vi "실습 2-8 Home 찾기.vi"   [LabVIEW 2014]
uses:
  <vilib>/Motion/FlexMotion/CustomControls/CustomControls.llb/AxisOrVectorSpace To Control.flx
  <vilib>/Motion/FlexMotion/FunctionsVIs/Trajectory.llb/Check Move Complete Status (8 axes).flx
types:
  T1 = enum16{"Home", "Index", "Center", "Forward Limit", "Reverse Limit", "Run Sequence"}
  T2 = typedef "AxisOrVectorSpace To Control.flx" = u16
  T3 = typedef "Board Id" = u8
  T4 = typedef "Resource Out (Enum).flx" = u16
  T5 = typedef "Bd Id Out" = u8
  T6 = typedef "AxisOrVectorSpaceControl To Control.flx" = u16
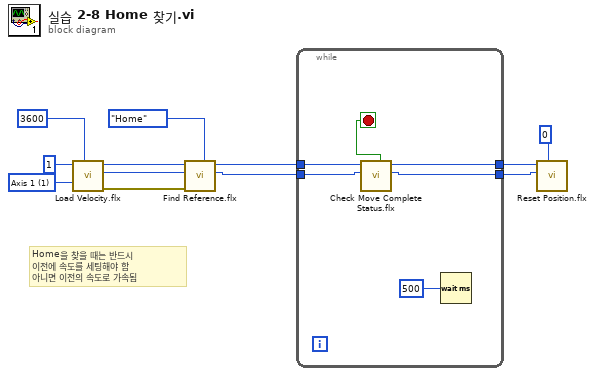
[diagram p0: block diagram]
diagram:
  w11 = T2 1 items=["Axis 1"=1, "Axis 2"=2, "Axis 3"=3, "Axis 4"=4, "Axis 5"=5, "Axis 6"=6, "Axis 7"=7, "Axis 8"=8, "Vector Space 1"=17, "Vector Space 2"=18, "Vector Space 3"=19, "Vector Space 4"=20] ("Axis or Vector Space")
  # "Home을 찾을 때는 반드시\n이전에 속도를 세팅해야 함\n아니면 이전의 속도로 가속됨"
  n1 = call <vilib>:"Load Velocity.flx"("Velocity (10000)"=3600, "Axis or Vector Space"=w11, "Board ID"=T3 1) -> ("error out"=w7:errorcluster, "Resource Output"=w8:T4, "Bd ID Out"=w9:T5)  [unwired: 4 in]
  n2 = call <vilib>:"Find Reference.flx"("Search Type"=T1."Home", "error in (no error)"=w7, "Axis or Vector Space"=w8, "Board ID"=w9) -> ("Axis or Vector Space Output"=w4:T6, "Bd ID Out"=w5:T5)  [unwired: 5 in, 1 out]
  n3 = while {
    tunnel: w5 -> [w18]
    tunnel: w4 -> [w17]
    tunnel: [w16] -> w3
    tunnel: [w15] -> w2
    stop <- w14 stop-if-true
    n4 = call-poly <vilib>:"Check Move Complete Status.flx"("Axis or Vector Space"=w17, "Board ID"=w18) -> ("Resource Output"=w15:T4, "Bd ID Out"=w16:T5, "Move Complete"=w14:bool)  [unwired: 4 in, 1 out]
    n5 = Wait (ms)(milliseconds to wait=u32 500 ("대기 시간(ms)")) -> ()  [unwired: 1 out]
  }
  n6 = call <vilib>:"Reset Position.flx"("Primary Reset Position (0)"=0, "Axis"=w2, "Board ID"=w3) -> ()  [unwired: 4 in, 3 out]
